vi "Send Stop Message to Nested Actors (SubVI).vi"(0 "Grayscale Enqueuers":refnum<class "Message Enqueuer.lvclass">[](array[class]), 11 "error in (no error)":errorcluster, 13 "Target Actor Enqueuers":T1=enum."Histogram") -> (15 "error out":errorcluster)   [LabVIEW 2016, in "Controller.lvlib" / "Controller.lvclass"]
uses:
  Controller.lvclass
  <vilib>/ActorFramework/Message Enqueuer/Message Enqueuer.lvclass
  Controls/List of Nested Actors.ctl
  <vilib>/ActorFramework/Message Enqueuer/Message Enqueuer.lvclass/Message Enqueuer.ctl
  <vilib>/ActorFramework/Message Enqueuer/Enqueue.vi
  Tests/Tests/Child Classes/Threshold Messages/Stop Threshold Actor Msg/Stop Threshold Actor Msg.lvclass
  C:/Program Files (x86)/National Instruments/LabVIEW 2016/vi.lib/ActorFramework/Message/Message.lvclass
  Tests/Tests/Child Classes/Grayscale Messages/Stop Grayscale Actor Msg/Stop Grayscale Actor Msg.lvclass
  Tests/Tests/Child Classes/Histogram Messages/Stop Histogram Actor Msg/Stop Histogram Actor Msg.lvclass
  UI/UI Messages/Stop UI Msg/Stop UI Msg.lvclass
  Image Acquisition/Image Acquisition Messages/Stop Acq Msg/Stop Acq Msg.lvclass
  <vilib>/ActorFramework/Message Priority Queue/Priority Enqueue.vi
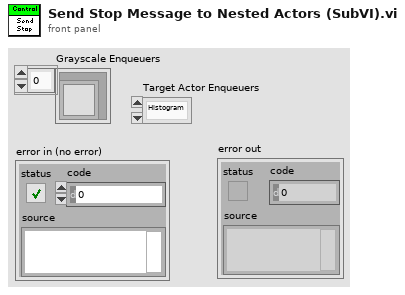
[diagram p1: front panel]
types:
  T1 = typedef "List of Nested Actors.ctl" = enum16{"Threshold", "Grayscale", "Histogram", "UI", "Acquisition"}
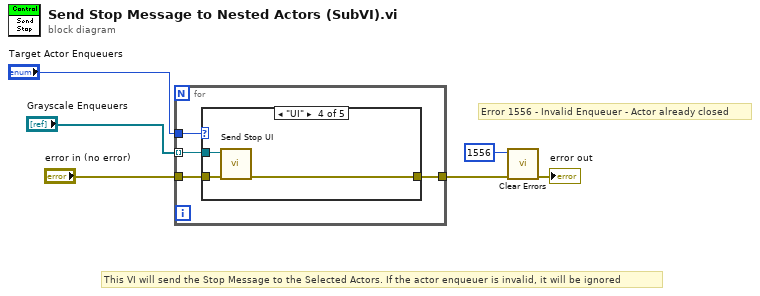
[diagram p0: block diagram]
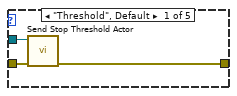
[diagram p2: hidden frame]
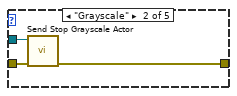
[diagram p3: hidden frame]
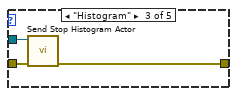
[diagram p4: hidden frame]
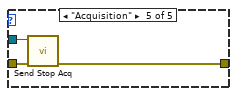
[diagram p5: hidden frame]
diagram:
  # "Error 1556 - Invalid Enqueuer - Actor already closed"
  # "This VI will send the Stop Message to the Selected Actors. If the actor enqueuer is invalid, it will be ignored"
  n1 = for {
    tunnel: "error in (no error)" -> [w10]
    tunnel: [w9] -> w4
    tunnel: "Grayscale Enqueuers" -> [w8] mode=indexing
    tunnel: "Target Actor Enqueuers" -> [w7]
    n2 = case shown="\"UI\"" w7 {
      tunnel: w10 -> [w13 w16 w19 w22 w25]
      tunnel: [w12 w15 w18 w21 w24] -> w9
      tunnel: w8 -> [w11 w14 w17 w20 w23]
      frame "Threshold", Default {
        n3 = call "Send Stop Threshold Actor.vi"("error in (no error)"=w13, "Message Enqueuer"=w11) -> ("error out"=w12:errorcluster)  [unwired: 8 in, 1 out]
      }
      frame "Grayscale" {
        n4 = call "Send Stop Grayscale Actor.vi"("error in (no error)"=w16, "Message Enqueuer"=w14) -> ("error out"=w15:errorcluster)  [unwired: 8 in, 1 out]
      }
      frame "Histogram" {
        n5 = call "Send Stop Histogram Actor.vi"("error in (no error)"=w19, "Message Enqueuer"=w17) -> ("error out"=w18:errorcluster)  [unwired: 8 in, 1 out]
      }
      frame "UI" {
        n6 = call "Send Stop UI.vi"("error in (no error)"=w22, "Message Enqueuer"=w20) -> ("error out"=w21:errorcluster)  [unwired: 8 in, 1 out]
      }
      frame "Acquisition" {
        n7 = call "Send Stop Acq.vi"("error in (no error)"=w25, "Message Enqueuer"=w23) -> ("error out"=w24:errorcluster)  [unwired: 8 in, 1 out]
      }
    }
  }
  n8 = call <vilib>:"Clear Errors.vi"("error in (no error)"=w4, "specific error code to clear (0: all)"=1556) -> ("error out"=→"error out":errorcluster)  [unwired: 4 in, 1 out]
